vi "PushPull.vi"() -> ()   [LabVIEW 2025]
uses:
  libzmq-v143-mt-4_3_6/ctls/SocketType.ctl
  zeromq/Receive_string.vi
  zeromq/Send_string.vi
  zeromq/Context.lvclass
  libzmq-v143-mt-4_3_6/LibZMQ.lvlib
  zeromq/Socket.lvclass
panel:
  out "data 2":string
  out "data":string
  out "error out 3":errorcluster
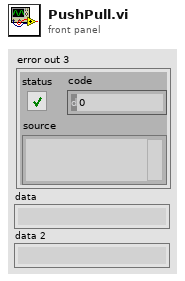
[diagram p1: front panel]
types:
  T1 = typedef "LibZMQ.lvlib/SocketType.ctl" = enum8{"PAIR", "PUB", "SUB", "REQ", "REP", "DEALER", "ROUTER", "PULL", "PUSH", "XPUB", "XSUB", "STREAM"}
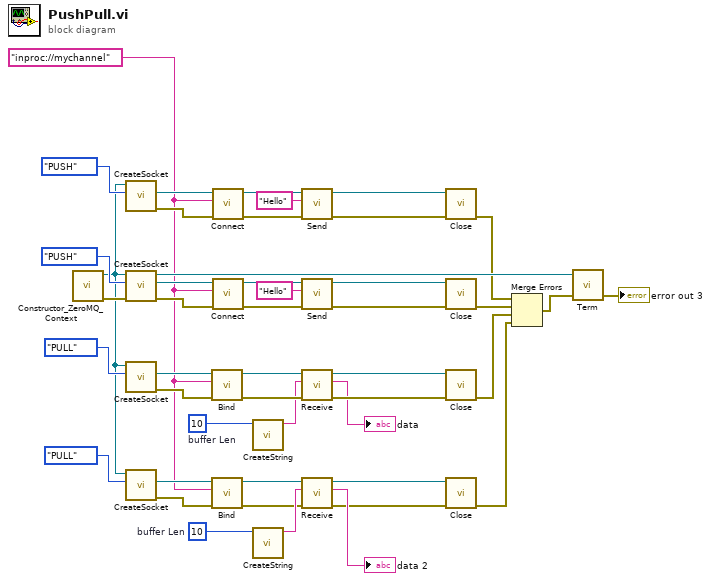
[diagram p0: block diagram]
diagram:
  w7 = 10  # buffer Len
  w39 = 10  # buffer Len
  w1 = "inproc://mychannel"
  n1 = call "Constructor_ZeroMQ_Context.vi"() -> ("error out"=w43:errorcluster, "context out"=w3:refnum<class "Context.lvclass">)  [unwired: 10 in]
  n2 = call "CreateSocket.vi"("Socket Type"=SocketType."PUSH", "context in"=w3) -> ("error out"=w22:errorcluster, "socket out"=w20:refnum<class "Socket.lvclass">)  [unwired: 7 in, 1 out]
  n3 = call "CreateSocket.vi"("error in"=w43, "Socket Type"=SocketType."PUSH", "context in"=w3) -> ("error out"=w31:errorcluster, "socket out"=w33:refnum<class "Socket.lvclass">, "context out"=w29:refnum<class "Context.lvclass">)  [unwired: 6 in]
  n4 = call "CreateSocket.vi"("Socket Type"=SocketType."PULL", "context in"=w3) -> ("error out"=w40:errorcluster, "socket out"=w41:refnum<class "Socket.lvclass">)  [unwired: 7 in, 1 out]
  n5 = call "CreateSocket.vi"("Socket Type"=SocketType."PULL", "context in"=w3) -> ("error out"=w6:errorcluster, "socket out"=w5:refnum<class "Socket.lvclass">)  [unwired: 7 in, 1 out]
  n6 = call "Bind.vi"("error in"=w40, "endpoint"=w1, "socket in"=w41) -> ("error out"=w37:errorcluster, "socket out"=w38:refnum<class "Socket.lvclass">)  [unwired: 7 in]
  n7 = call "Bind.vi"("error in"=w6, "endpoint"=w1, "socket in"=w5) -> ("error out"=w9:errorcluster, "socket out"=w8:refnum<class "Socket.lvclass">)  [unwired: 7 in]
  n8 = call "Connect.vi"("error in"=w22, "endpoint"=w1, "socket in"=w20) -> ("error out"=w23:errorcluster, "socket out"=w21:refnum<class "Socket.lvclass">)  [unwired: 7 in]
  n9 = call "Connect.vi"("error in"=w31, "endpoint"=w1, "socket in"=w33) -> ("error out"=w30:errorcluster, "socket out"=w32:refnum<class "Socket.lvclass">)  [unwired: 7 in]
  n10 = call "CreateString.vi"("length"=w39) -> ("string"=w15:string)  [unwired: 10 in]
  n11 = call "CreateString.vi"("length"=w7) -> ("string"=w12:string)  [unwired: 10 in]
  n12 = call-poly "Send.vi"("error in"=w23, "data"="Hello", "socket in"=w21) -> ("error out"=w19:errorcluster, "socket out"=w18:refnum<class "Socket.lvclass">)  [unwired: 7 in]
  n13 = call-poly "Send.vi"("error in"=w30, "data"="Hello", "socket in"=w32) -> ("error out"=w34:errorcluster, "socket out"=w35:refnum<class "Socket.lvclass">)  [unwired: 7 in]
  n14 = call-poly "Receive.vi"("error in"=w37, "buf in"=w15, "socket in"=w38) -> ("error out"=w27:errorcluster, "data"=→"data":string, "socket out"=w28:refnum<class "Socket.lvclass">)  [unwired: 6 in]
  n15 = call-poly "Receive.vi"("error in"=w9, "buf in"=w12, "socket in"=w8) -> ("error out"=w11:errorcluster, "data"=→"data 2":string, "socket out"=w10:refnum<class "Socket.lvclass">)  [unwired: 6 in]
  n16 = call "Close.vi"("error in"=w19, "socket"=w18) -> ("error out"=w16:errorcluster)  [unwired: 9 in]
  n17 = call "Close.vi"("error in"=w34, "socket"=w35) -> ("error out"=w44:errorcluster)  [unwired: 9 in]
  n18 = call "Close.vi"("error in"=w27, "socket"=w28) -> ("error out"=w26:errorcluster)  [unwired: 9 in]
  n19 = call "Close.vi"("error in"=w11, "socket"=w10) -> ("error out"=w2:errorcluster)  [unwired: 9 in]
  n20 = Merge Errors(w16, w44, w26, w2) -> (w45:errorcluster)
  n21 = call "Term.vi"("error in"=w45, "context in"=w29) -> ("error out"=→"error out 3":errorcluster)  [unwired: 3 in]
